vi "Find Key Values.vi"() -> ()   [LabVIEW 2015]
uses:
  <vilib>/Utility/config.llb/Config Data RefNum.ctl
  <vilib>/regexp/Match Regular Expression.xnode
  <vilib>/Utility/config.llb/NI_LVConfig.lvlib
panel:
  out "refnum":T1
  in  "Search":string
  out "Preferences":string[][](array[string])
  in  "stop":bool
  in  "Possible Choices":i32(ring)=1 items=["Hue1", "Hue2"]
  out "Value":string="NA"
  out "Key":string="NA"
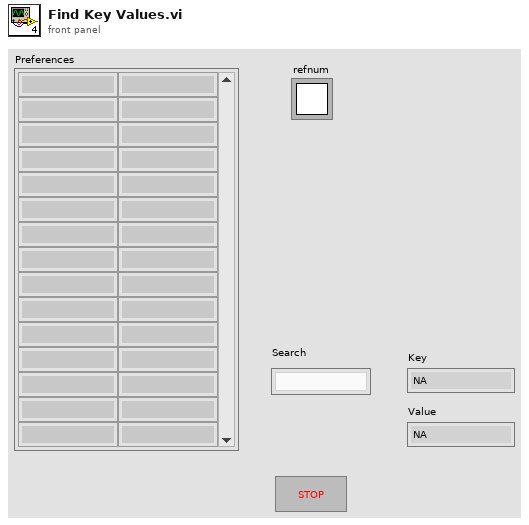
[diagram p1: front panel]
types:
  T1 = typedef "NI_LVConfig.lvlib/Config Data RefNum.ctl" = refnum<k1>
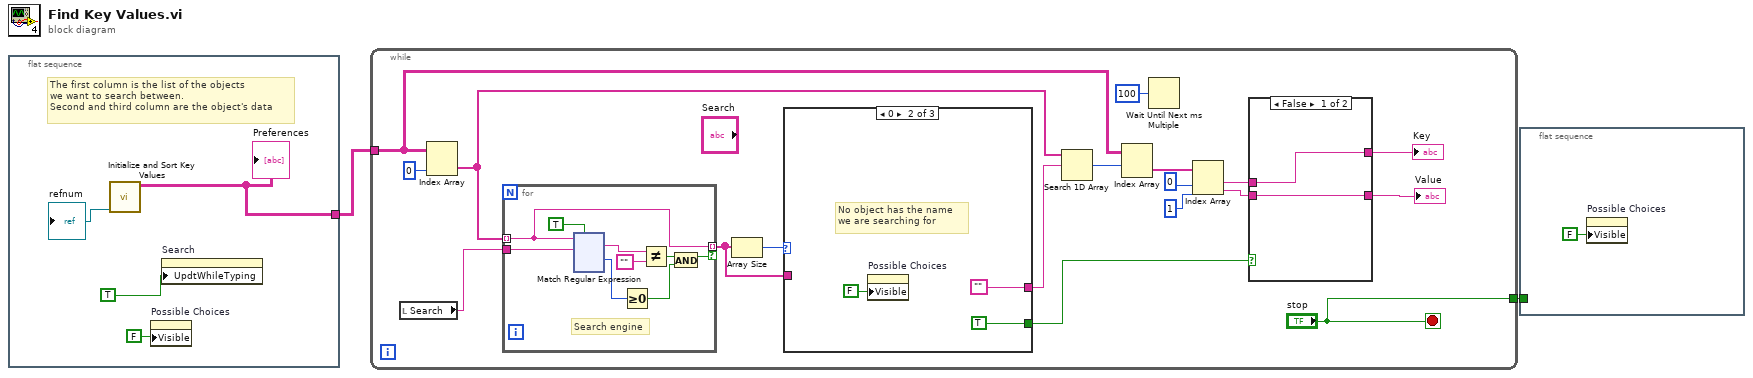
[diagram p0: block diagram]
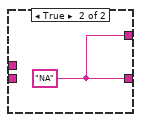
[diagram p2: hidden frame]
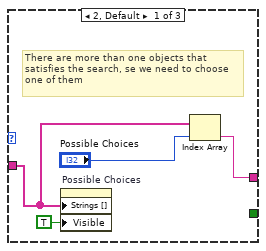
[diagram p3: hidden frame]
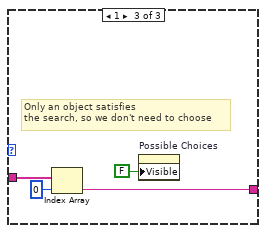
[diagram p4: hidden frame]
diagram:
  n1 = flat-sequence {
    tunnel: [w4] -> w2
    frame #0 {
      # "The first column is the list of the objects \nwe want to search between.\nSecond and third column are the object's data"
      n2 = call "Initialize and Sort Key Values.vi"() -> ("refnum"=→"refnum":T1, "Preferences"=w4:string[][])  [unwired: 10 in]
      "Preferences" <- w4
      n3 = property on="Possible Choices" class="Ring (strict)"("Visible"=FALSE) -> ()  [unwired: 2 in, 2 out]
      n4 = property on="Search" class="Str"("UpdtWhileTyping"=TRUE ("Update While Typing?")) -> ()  [unwired: 2 in, 2 out]
    }
  }
  n5 = while {
    tunnel: w2 -> [w22]
    tunnel: ["stop"] -> w1
    stop <- "stop" stop-if-true
    n6 = local read "Search"() -> (w9:string)
    n7 = Index Array(array=w22, index (col)=0 ("disabled index (col)")) -> (element=w19:string[])  [unwired: 1 in]
    n8 = for {
      tunnel: w9 -> [w47]
      tunnel: w19 -> [w43] mode=indexing
      tunnel: [w43] -> w20 mode=indexing if=w41
      # "Search engine"
      n9 = xnode "Match Regular Expression"("input string"=w43, "regular expression"=w47, "ignore case? (F)"=TRUE) -> ("whole match"=w45:string, "offset past match"=w42:i32)  [unwired: 3 in, 3 out]
      n10 = Greater Or Equal To 0?(x=w42) -> (x >= 0?=w40:bool)
      n11 = Not Equal?(x=w45, y="") -> (x != y?=w44:bool)
      n12 = And(x=w44, y=w40) -> (x .and. y?=w41:bool)
    }
    n13 = Array Size(array=w20) -> (size(s)=w21:i32)
    n14 = case shown="0" w21 {
      tunnel: w20 -> [w31 _ w38]
      tunnel: [w30 "" w36] -> w18
      tunnel: [_ TRUE ("Visible") _] -> w12
      frame 2, Default {
        # "There are more than one objects that\nsatisfies the search, se we need to choose\none of them"
        n15 = property on="Possible Choices" class="Ring (strict)"("Strings []"=w31, "Visible"=TRUE) -> ()  [unwired: 2 in, 2 out]
        n16 = Index Array(array=w31, index="Possible Choices") -> (element=w30:string)
      }
      frame 0 {
        # "No object has the name \nwe are searching for"
        n17 = property on="Possible Choices" class="Ring (strict)"("Visible"=FALSE) -> ()  [unwired: 2 in, 2 out]
      }
      frame 1 {
        # "Only an object satisfies\nthe search, so we don't need to choose"
        n18 = Index Array(array=w38, index=0) -> (element=w36:string)
        n19 = property on="Possible Choices" class="Ring (strict)"("Visible"=FALSE) -> ()  [unwired: 2 in, 2 out]
      }
    }
    n20 = Search 1D Array(1D array=w19, element=w18) -> (index of element=w17:i32)  [unwired: 1 in]
    n21 = Index Array(array=w22, index (row)=w17) -> (element=w15:string[])  [unwired: 1 in]
    n22 = Wait Until Next ms Multiple(millisecond multiple=u32 100) -> ()  [unwired: 1 out]
    n23 = Index Array(array=w15, index #1=0 ("index"), index #2=1 ("index")) -> (element #1=w11:string, element #2=w10:string)
    n24 = case shown="False" w12 {
      tunnel: [w26 w27] -> w7
      tunnel: w11 -> [w26 _]
      tunnel: [w25 w27] -> w8
      tunnel: w10 -> [w25 _]
      frame False {
      }
      frame True {
        w27 = "NA" ("String")
      }
    }
    "Value" <- w8
    "Key" <- w7
  }
  n25 = flat-sequence {
    tunnel: w1 -> [_]
    frame #0 {
      n26 = property on="Possible Choices" class="Ring (strict)"("Visible"=FALSE) -> ()  [unwired: 2 in, 2 out]
    }
  }
